vi "ErrorsFGV.vi"(8 "CriticalErrorIn":errorcluster, 9 "InternalErrorIn":errorcluster, 10 "Reset?":bool) -> (0 "CriticalErrorOut":errorcluster, 1 "InternalErrorOut":errorcluster, 2 "GetCriticalError":errorcluster, 3 "GetInternalError":errorcluster)   [LabVIEW 2019]
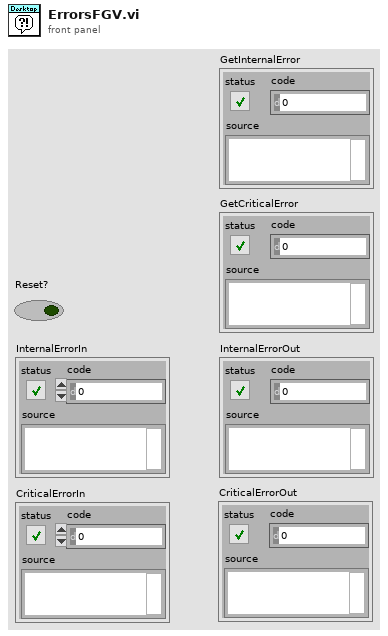
[diagram p1: front panel]
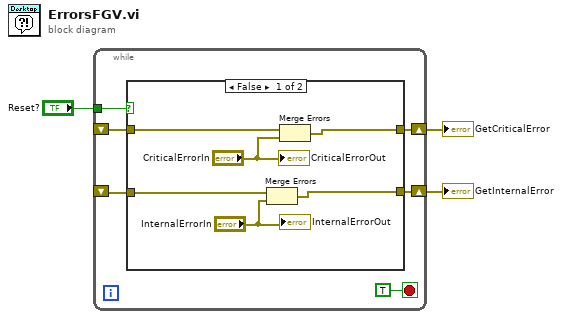
[diagram p0: block diagram]
diagram:
  n1 = while {
    shift-right: [w8] -> w2
    shift-left: _ -> [w7]
    tunnel: "Reset?" -> [w6]
    shift-right: [w4] -> w1
    shift-left: _ -> [w5]
    stop <- TRUE stop-if-true
    n2 = case shown="False" w6 {
      tunnel: [w15 _] -> w8
      tunnel: w7 -> [w12 _]
      tunnel: w5 -> [w13 _]
      tunnel: [w14 _] -> w4
      frame False {
        n3 = Merge Errors(w13, "InternalErrorIn") -> (w14:errorcluster)
        n4 = Merge Errors(w12, "CriticalErrorIn") -> (w15:errorcluster)
        "InternalErrorOut" <- "InternalErrorIn"
        "CriticalErrorOut" <- "CriticalErrorIn"
      }
      frame True {
      }
    }
  }
  "GetCriticalError" <- w2
  "GetInternalError" <- w1
